vi "Pre Launch Init.vi"(11 "Feeder Pressure in":refnum<class "Feeder Pressure.lvclass">) -> (0 "error out":errorcluster, 3 "Feeder Pressure out":refnum<class "Feeder Pressure.lvclass">)   [LabVIEW 2018, in "Pressure Actor.lvlib" / "Feeder Pressure.lvclass"]
doc: "(<B>Filename</B>: Actor Framework.lvlib:Actor.lvclass:Pre Launch Init.vi)\n\nDefines behavior that occurs after the Launch Nested Actor method is invoked but before the actor's Actor Core method begins running.\n\nBy default, this method does nothing. A descendant class may override it to define behavior."
uses:
  Feeder Pressure.lvclass
  Feeder Pressure.lvclass/Feeder Pressure.ctl
  Pressure/Pressure.lvclass
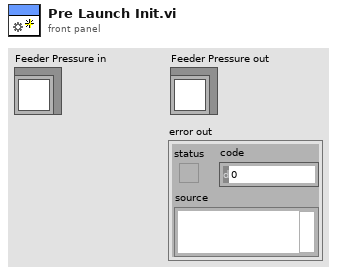
[diagram p1: front panel]
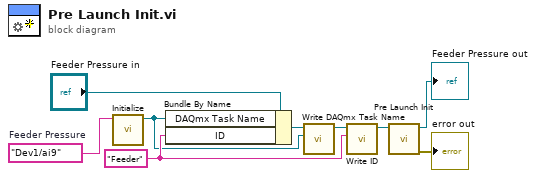
[diagram p0: block diagram]
diagram:
  w1 = tag "Dev1/ai9"  # Feeder Pressure
  w4 = "Feeder" ("ID")
  n1 = call "Initialize.vi"("physical channels"=w1) -> ("task out"=w2:refnum<k21>)  [unwired: 9 in, 1 out]
  n2 = Bundle By Name(cluster="Feeder Pressure in", "DAQmx Task Name"=w2, "ID"=w4) -> (w6:refnum<class "Feeder Pressure.lvclass">)
  n3 = call-dynamic "Write DAQmx Task Name.vi"("DAQmx Task Name"=w2, "Pressure in"=w6) -> ("Pressure out"=w5:refnum<class "Feeder Pressure.lvclass">)  [unwired: 8 in, 1 out]
  n4 = call-dynamic "Write ID.vi"("ID"=w4, "Pressure in"=w5) -> ("Pressure out"=w3:refnum<class "Feeder Pressure.lvclass">)  [unwired: 8 in, 1 out]
  n5 = call-parent "Pre Launch Init.vi"("Pressure in"=w3) -> ("error out"=→"error out":errorcluster, "Pressure out"=→"Feeder Pressure out":refnum<class "Feeder Pressure.lvclass">)  [unwired: 9 in]
